vi "convert from unicode.vi"(11 "UTF8 String":string) -> (3 "System String":string)   [LabVIEW 2013, in "lvnano.lvlib"]
uses:
  lvnano.lvlib
  lvnanomsg.dll
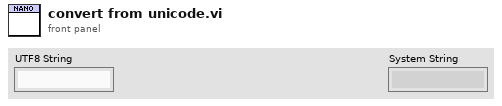
[diagram p1: front panel]
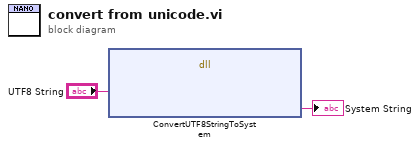
[diagram p0: block diagram]
diagram:
  n1 = dll-call lib="C:/Users/Daniel/Documents/nanomsg/lvnano/lvnanomsg.*" fn="ConvertUTF8StringToSystem"("UTF8 String"="UTF8 String") -> ("System String"=→"System String":string)  [unwired: 6 in, 2 out]
